vi "CalculateTime.vi"(1 "distance":dbl) -> (0 "time min:s:ms":string)   [LabVIEW 2020]
doc: "Returns information about time needed for data to flow depending on distance (d)."
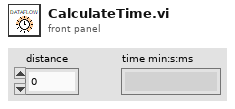
[diagram p1: front panel]
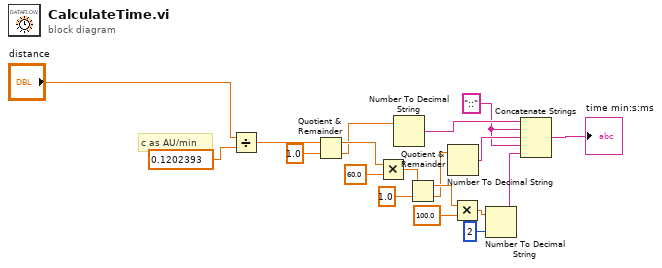
[diagram p0: block diagram]
diagram:
  w6 = "::" ("string")
  # "c as AU/min"
  n1 = Divide(x="distance", y=0.1202393) -> (x/y=w3:dbl)
  n2 = Quotient & Remainder(x=w3, y=1.0) -> (x-y*floor(x/y)=w10:dbl, floor(x/y)=w9:dbl)
  n3 = Multiply(x=w10, y=60.0) -> (x*y=w13:dbl)
  n4 = Number To Decimal String(number=w9) -> (decimal integer string=w8:string)  [unwired: 1 in]
  n5 = Quotient & Remainder(x=w13, y=1.0) -> (x-y*floor(x/y)=w15:dbl, floor(x/y)=w14:dbl)
  n6 = Number To Decimal String(number=w14) -> (decimal integer string=w11:string)  [unwired: 1 in]
  n7 = Multiply(x=w15, y=100.0) -> (x*y=w17:dbl)
  n8 = Number To Decimal String(number=w17, width (-)=i16 2) -> (decimal integer string=w18:string)
  n9 = Concatenate Strings(w8, w6, w11, w6, w18) -> (→"time min:s:ms":string)
